vi "Init.vi"(8 "error in (no error)":errorcluster, 9 "Config File Path":path=path "", 10 "Name":string, 11 "Mock Job Handler In":refnum<class "Mock Job Handler.lvclass">) -> (0 "error out":errorcluster, 3 "Mock Job Handler Out":refnum<class "Mock Job Handler.lvclass">)   [LabVIEW 2020, in "Mock Job Handler.lvclass"]
doc: "Initialize the class and creates necessary references. Anything initialized here is released in the Clear.vi method."
uses:
  Mock Job Handler.lvclass
  Processes/People/Process Job/Job Handler.lvclass
  Mock Job Handler.lvclass/Mock Job Handler.ctl
  <vilib>/Astemes/Triarc Framework/Base/Base.lvclass
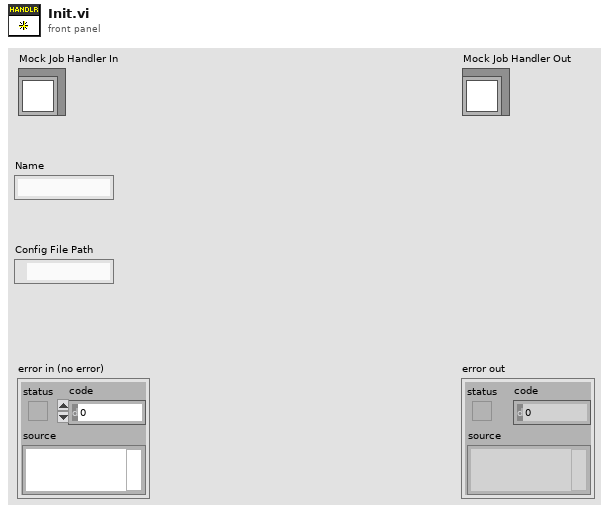
[diagram p1: front panel]
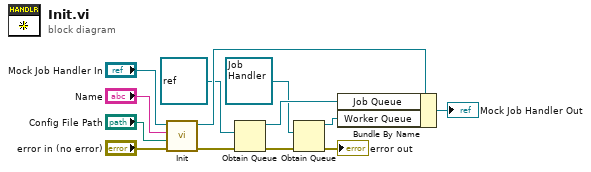
[diagram p0: block diagram]
diagram:
  n1 = call-parent "Init.vi"("error in (no error)"="error in (no error)", "Config File Path"="Config File Path", "Name"="Name", "Base In"="Mock Job Handler In") -> ("error out"=w5:errorcluster, "Base Out"=w13:refnum<class "Mock Job Handler.lvclass">)  [unwired: 6 in]
  n2 = Obtain Queue(element data type=refnum<class> refnum ("LabVIEW Object"), error in (no error)=w5) -> (queue out=w6:refnum<queue>, error out=w2:errorcluster)  [unwired: 3 in, 1 out]
  n3 = Obtain Queue(element data type=refnum<class "Job Handler.lvclass"> refnum ("Job Handler.lvclass"), error in (no error)=w2) -> (queue out=w3:refnum<queue>, error out=→"error out":errorcluster)  [unwired: 3 in, 1 out]
  n4 = Bundle By Name(cluster=w13, "Job Queue"=w6, "Worker Queue"=w3) -> (→"Mock Job Handler Out":refnum<class "Mock Job Handler.lvclass">)
